vi "5302GetOscFreq.vi"(8 "error in (no error)":errorcluster, 11 "VISA Resource Name":refnum<visa-resource-name>) -> (0 "error out":errorcluster, 1 "data string":string, 2 "Osc Freq":dbl format="%.4f", 3 "VISA Resource Name Out":refnum<visa-resource-name>)   [LabVIEW 2015]
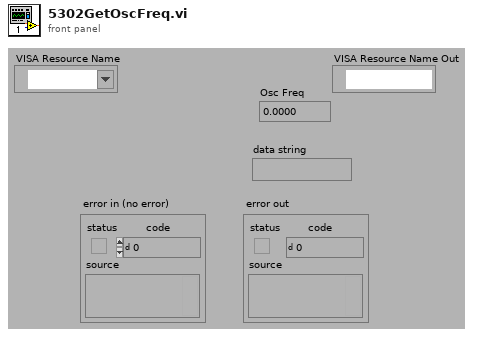
[diagram p1: front panel]
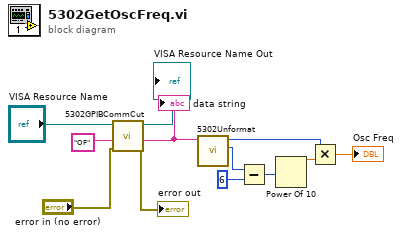
[diagram p0: block diagram]
diagram:
  n1 = call "5302GPIBCommCut.vi"("error in (no error)"="error in (no error)", "data string in"="OF" ("data string"), "VISA Resource Name"="VISA Resource Name") -> ("error out"=→"error out":errorcluster, "data string out"=w3:string, "VISA Resource Name Out"=→"VISA Resource Name Out":refnum<visa-resource-name>)  [unwired: 2 in, 4 out]
  "data string" <- w3
  n2 = call "5302Unformat.vi"("Data String"=w3) -> ("Numeric 2"=w5:i32, "Numeric 1"=w4:i32)  [unwired: 9 out]
  n3 = Subtract(x=w5, y=6) -> (x-y=w8:i32)
  n4 = Power Of 10(x=w8) -> (10^x=w7:dbl)
  n5 = Multiply(x=w4, y=w7) -> (x*y=→"Osc Freq":dbl)
